vi "publicador.vi"() -> ()   [LabVIEW 2020]
uses:
  <vilib>/LabVIEW Open Source Project/MQTT Client/Client class/Client.lvclass
  C:/Program Files (x86)/National Instruments/LabVIEW 2020/vi.lib/LabVIEW Open Source Project/MQTT Connection/MQTT_Base/Base Class/MQTT_Base.lvclass
  <vilib>/LabVIEW Open Source Project/MQTT Client/Client class/Client.lvclass/Client.ctl
  <vilib>/LabVIEW Open Source Project/MQTT Connection/MQTT_Base/Base Class/MQTT_Base.lvclass/MQTT_Base.ctl
  <vilib>/LabVIEW Open Source Project/MQTT TCP Connection/MQTT_TCP/Connection/TCPConnection.lvclass
  C:/Program Files (x86)/National Instruments/LabVIEW 2020/vi.lib/LabVIEW Open Source Project/Connection/Connection/Connection.lvclass
  <vilib>/ErrorRing/Error Ring.xnode
  <vilib>/LabVIEW Open Source Project/MQTT Control Packets/Control Packets/PUBLISH/PUBLISH.lvclass
  <vilib>/LabVIEW Open Source Project/MQTT Connection/MQTT_Base/Base Class/MQTT_Base.lvclass
  <vilib>/LabVIEW Open Source Project/Connection/Connection.LocalQueue/Connection.LocalQueue.lvclass
  <vilib>/LabVIEW Open Source Project/Connection/Connection/Connection.lvclass
panel:
  out "variant":variant
  out "Client out":refnum<class "Client.lvclass">
  in  "Thermometer":dbl(slide) scale=0.0..100.0
  in  "Connection":bool
  in  "Stop Client":bool
  out "Published":bool
  out "Waveform Chart":dbl(graph)
  out "last error":errorcluster
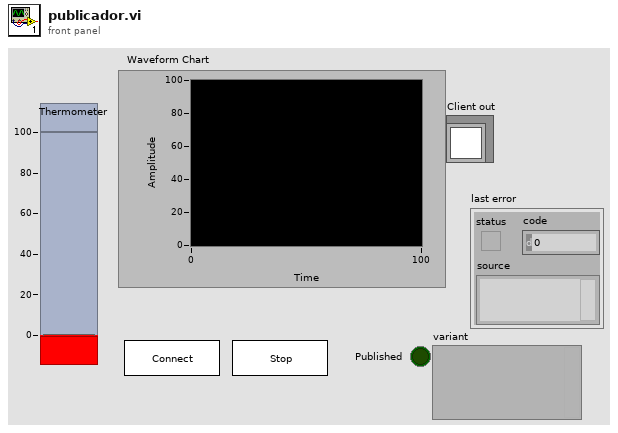
[diagram p1: front panel]
types:
  T1 = typedef "MQTT Client.lvlib/Client.lvclass/Public Events -- cluster.ctl" = cluster{"Connection Status":refnum<user-event>, "Connected":refnum<user-event>, "Application Message":refnum<user-event>}
  T2 = typedef "MQTT Base.lvlib/MQTT_Base.lvclass/Public Events -- cluster.ctl" = cluster{"Stop Event":refnum<user-event>, "Error Event":refnum<user-event>, "Inbound Message":refnum<user-event>}
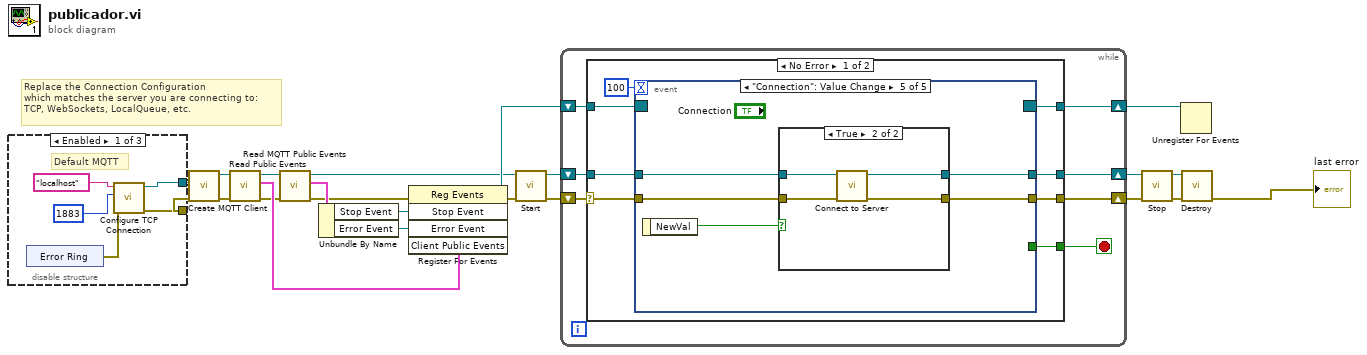
[diagram p0: block diagram]
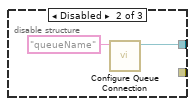
[diagram p2: hidden frame]
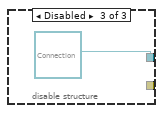
[diagram p3: hidden frame]
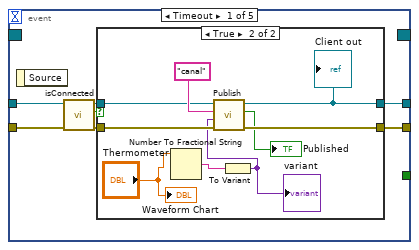
[diagram p4: hidden frame]
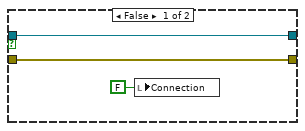
[diagram p5: hidden frame]
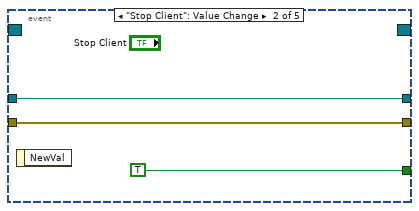
[diagram p6: hidden frame]
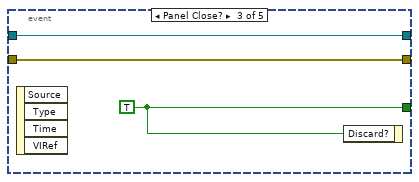
[diagram p7: hidden frame]
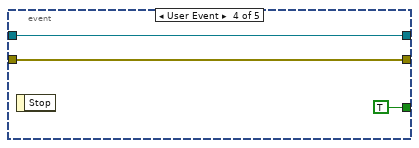
[diagram p8: hidden frame]
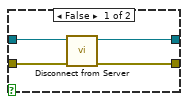
[diagram p9: hidden frame]
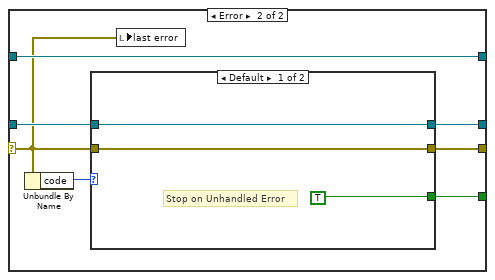
[diagram p10: hidden frame]
diagram:
  # "Replace the Connection Configuration\nwhich matches the server you are connecting to:\nTCP, WebSockets, LocalQueue, etc."
  n1 = disable-structure shown="Enabled" {
    disable-tunnel: [w26 w30 refnum<class "Connection.lvclass"> refnum ("Connection Configuration")] -> w22
    disable-tunnel: [w27 _ _] -> w1
    frame Enabled {
      # "Default MQTT"
      n2 = xnode "Error Ring"() -> ("error out"=w23:errorcluster)
      n3 = call <vilib>:"Configure TCP Connection.vi"("error in (no error)"=w23, "remote port (80)"=u16 1883, "address (localhost)"="localhost") -> ("error out"=w27:errorcluster, "TCPConnection"=w26:refnum<class "TCPConnection.lvclass">)  [unwired: 7 in]
    }
    frame Disabled {
      n4 = call <vilib>:"Configure Queue Connection.vi"("Queue Name"="queueName") -> ("Connection.LocalQueue"=w30:refnum<class "Connection.LocalQueue.lvclass">)  [unwired: 9 in, 1 out]
    }
    frame Disabled {
    }
  }
  n5 = call <vilib>:"Create MQTT Client.vi"("error in (no error)"=w1, "Connection Configuration"=w22) -> ("error out"=w4:errorcluster, "Client out"=w2:refnum<class "Client.lvclass">)  [unwired: 8 in]
  n6 = call <vilib>:"Read Public Events.vi"("error in (no error)"=w4, "Client in"=w2) -> ("error out"=w5:errorcluster, "Client Public Events"=w7:T1, "Client out"=w3:refnum<class "Client.lvclass">)  [unwired: 7 in]
  n7 = call <vilib>:"Read MQTT Public Events.vi"("error in (no error)"=w5, "MQTT_Base in"=w3) -> ("error out"=w6:errorcluster, "MQTT Public Events"=w14:T2, "MQTT_Base out"=w9:refnum<class "Client.lvclass">)  [unwired: 7 in]
  n8 = Unbundle By Name(w14) -> ("Stop Event"=w12:refnum<user-event>, "Error Event"=w13:refnum<user-event>)
  n9 = register-events(error in=w6, w12, w13, w7) -> (reference out=w10:refnum<event-registration>, error out=w8:errorcluster)  [unwired: 1 in]
  n10 = call <vilib>:"Start.vi"("error in (no error)"=w8, "MQTT_Base in"=w9) -> ("error out"=w20:errorcluster, "MQTT_Base out"=w19:refnum<class "Client.lvclass">)  [unwired: 7 in, 1 out]
  n11 = while {
    shift-right: [w37] -> w11
    shift-left: w10 -> [w38]
    shift-right: [w34] -> w16
    shift-left: w19 -> [w35]
    shift-right: [w36] -> w18
    shift-left: w20 -> [w32]
    stop <- w33 stop-if-true
    n12 = case shown="No Error" w32 {
      selector: w32 -> [w39 w88]
      tunnel: w38 -> [w46 w94]
      tunnel: [w45 w94] -> w37
      tunnel: [w44 w90] -> w36
      tunnel: w35 -> [w42 w92]
      tunnel: [w41 w91] -> w34
      tunnel: [w40 w89] -> w33
      frame No Error {
        n13 = event shown="[4] \"Connection\": Value Change" {
          selector: w46 -> [_ _ _ _ _]
          dyn-events: [_ _ _ _ _] -> w45
          timeout: 100 -> [_ _ _ _ _]
          tunnel: w39 -> [w49 w67 w69 w74 w75]
          tunnel: [w52 w67 w69 w74 w76] -> w44
          tunnel: [_ TRUE w71 TRUE _] -> w40
          tunnel: w42 -> [w51 w68 w70 w72 w79]
          tunnel: [w53 w68 w70 w72 w77] -> w41
          event Timeout {
            n14 = event-data() -> ()  [unwired: 1 in, 1 out]
            n15 = call <vilib>:"isConnected.vi"("error in (no error)"=w49, "Client in"=w51) -> ("error out"=w48:errorcluster, "connected"=w47:bool, "Client out"=w50:refnum<class "Client.lvclass">)  [unwired: 7 in]
            n16 = case shown="True" w47 {
              tunnel: [w56 w64] -> w53
              tunnel: [w55 w63] -> w52
              tunnel: w50 -> [w56 w61]
              tunnel: w48 -> [w55 w60]
              frame False {
                n17 = local write "Connection"(FALSE ("Connection")) -> ()
              }
              frame True {
                n18 = Number To Fractional String(number="Thermometer") -> (F-format string=w58:string)  [unwired: 3 in]
                n19 = To Variant(anything=w58) -> (Variant=w57:variant)
                "variant" <- w57
                n20 = call <vilib>:"Publish.vi"("error in (no error)"=w60, "Payload"=w57, "Topic Name (empty: Payload name)"="canal", "Client in"=w61) -> ("error out"=w63:errorcluster, "Published"=→"Published":bool, "Client out"=w64:refnum<class "Client.lvclass">)  [unwired: 5 in]
                "Client out" <- w64
                "Waveform Chart" <- "Thermometer"
              }
            }
          }
          event "Stop Client": Value Change {
            n21 = event-data() -> ()  [unwired: 1 in, 1 out]
          }
          event Panel Close? {
            w71 = TRUE
            n22 = event-data() -> ()  [unwired: 1 in, 4 out]
            n23 = event-data("Discard?"=w71) -> ()  [unwired: 1 in, 1 out]
          }
          event User Event {
            n24 = event-data() -> ()  [unwired: 1 in, 1 out]
          }
          event "Connection": Value Change {
            n25 = event-data() -> ("NewVal"=w78:bool)  [unwired: 1 in]
            n26 = case shown="True" w78 {
              tunnel: w79 -> [w83 w87]
              tunnel: [w82 w84] -> w77
              tunnel: [w81 w85] -> w76
              tunnel: w75 -> [w80 w86]
              frame False {
                n27 = call <vilib>:"Disconnect from Server.vi"("error in (no error)"=w80, "Client in"=w83) -> ("error out"=w81:errorcluster, "Client out"=w82:refnum<class "Client.lvclass">)  [unwired: 7 in, 1 out]
              }
              frame True {
                n28 = call <vilib>:"Connect to Server.vi"("error in (no error)"=w86, "Client in"=w87) -> ("error out"=w85:errorcluster, "Client out"=w84:refnum<class "Client.lvclass">)  [unwired: 6 in, 2 out]
              }
            }
          }
        }
      }
      frame Error {
        n29 = Unbundle By Name(w88) -> ("code"=w93:i32)
        n30 = case shown="Default" w93 {
          tunnel: w92 -> [w97 w98]
          tunnel: [w97 w98] -> w91
          tunnel: w88 -> [w96 _]
          tunnel: [w96 _] -> w90
          tunnel: [TRUE _] -> w89
          frame Default {
            # "Stop on Unhandled Error"
          }
          frame 56, 63, 66 {
            # "Disconnected"
          }
        }
        n31 = local write "last error"(w88) -> ()
      }
    }
  }
  n32 = call <vilib>:"Stop.vi"("error in (no error)"=w18, "MQTT_Base in"=w16) -> ("error out"=w17:errorcluster, "MQTT_Base out"=w15:refnum<class "Client.lvclass">)  [unwired: 7 in, 1 out]
  n33 = Unregister For Events(event registration refnum=w11) -> ()  [unwired: 1 in, 1 out]
  n34 = call <vilib>:"Destroy.vi"("error in (no error)"=w17, "MQTT_Base in"=w15) -> ("error out"=→"last error":errorcluster)  [unwired: 8 in, 1 out]
